vi "SkipForward.vi"(8 "error in (no error)":errorcluster, 10 "Message Queues in":T2, 11 "UI Refs in":T1) -> (0 "error out":errorcluster, 2 "Message Queues out":T2, 3 "UI Refs out":T1)   [LabVIEW 2015]
uses:
  support/Message Queue/All Message Queues.ctl
  support/Message Queue/Message Cluster.ctl
  Controls & Type Defs/UI Data.ctl
  Controls & Type Defs/SongDetails.ctl
  support/Message Queue/Enqueue Message (Single).vi
  support/Message Queue/Message Queue.lvlib
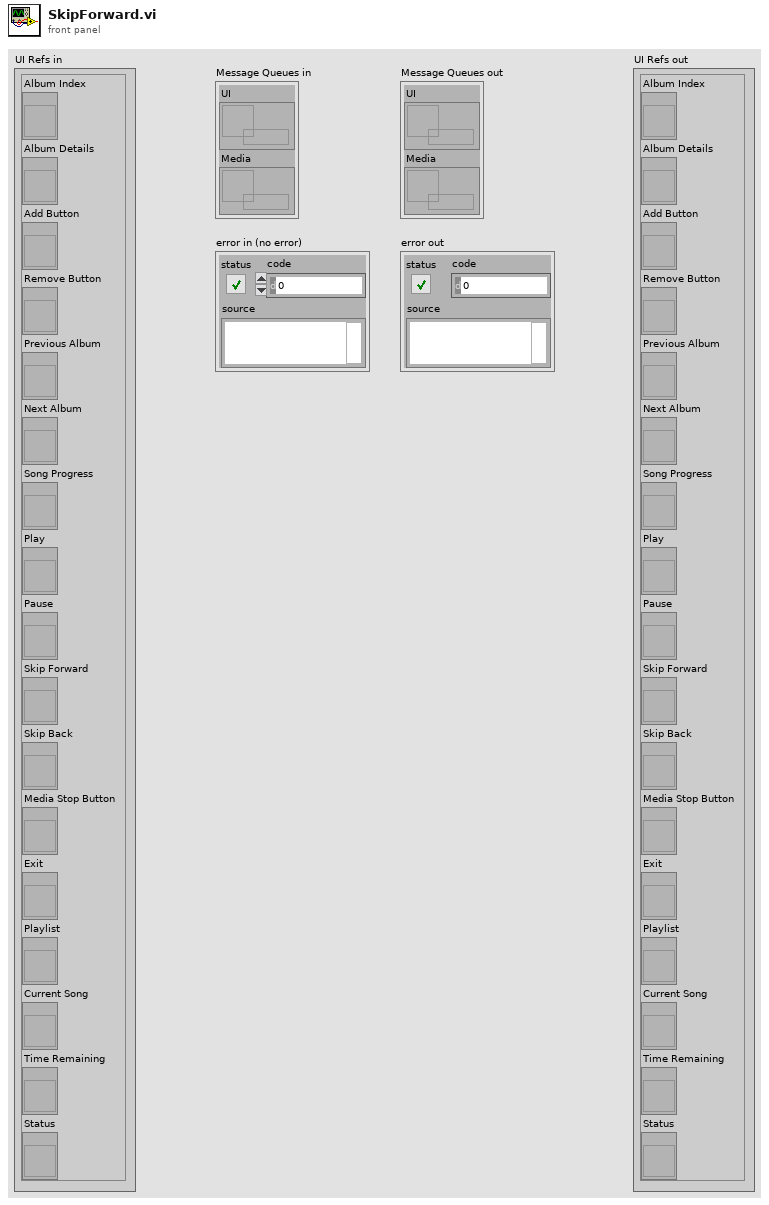
[diagram p1: front panel]
types:
  T1 = typedef "UI Data.ctl" = cluster{"Album Index":refnum<vi>, "Album Details":refnum<vi>, "Add Button":refnum<vi>, "Remove Button":refnum<vi>, "Previous Album":refnum<vi>, "Next Album":refnum<vi>, "Song Progress":refnum<vi>, "Play":refnum<vi>, "Pause ":refnum<vi>, "Skip Forward":refnum<vi>, "Skip Back":refnum<vi>, "Media Stop Button":refnum<vi>, "Exit":refnum<vi>, "Playlist":refnum<vi>, "Current Song":refnum<vi>, "Time Remaining":refnum<vi>, "Status":refnum<vi>}
  T2 = typedef "Message Queue.lvlib/All Message Queues.ctl" = cluster{"UI":refnum<queue>, "Media":refnum<queue>}
  T3 = typedef "SongDetails.ctl" = cluster{"Artist - Song Name":string, "Duration":string}
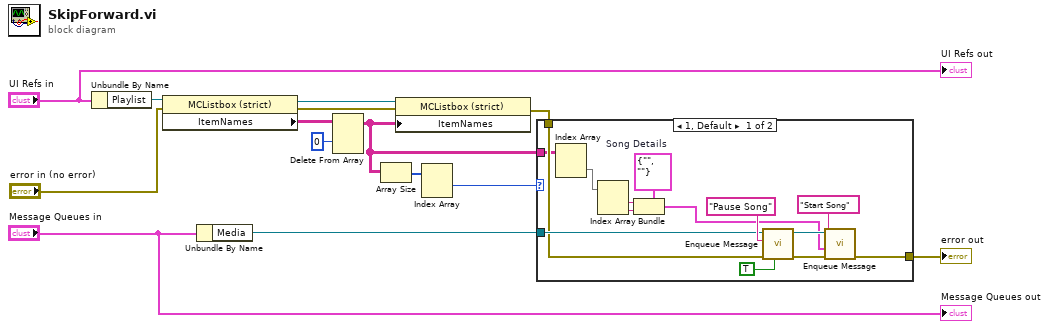
[diagram p0: block diagram]
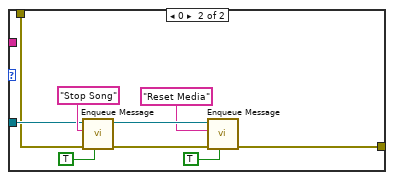
[diagram p2: hidden frame]
diagram:
  n1 = Unbundle By Name("UI Refs in") -> ("Playlist"=w14:refnum<vi>)
  n2 = property class="MCListbox (strict)"(reference=w14, error in="error in (no error)") -> (reference out=w11:refnum<vi>, error out=w10:errorcluster, "ItemNames"=w13:string[][])
  n3 = Unbundle By Name("Message Queues in") -> ("Media"=w9:refnum<queue>)
  n4 = Delete From Array(array=w13, index (row)=0) -> (array with subset deleted=w4:string[][])  [unwired: 2 in, 1 out]
  n5 = Array Size(array=w4) -> (size(s)=w3:i32[])
  n6 = property class="MCListbox (strict)"(reference=w11, error in=w10, "ItemNames"=w4) -> (error out=w8:errorcluster)  [unwired: 1 out]
  n7 = Index Array(array=w3) -> (element #1=w2:i32)  [unwired: 2 in, 1 out]
  n8 = case shown="1, Default" w2 {
    tunnel: w9 -> [w23 w36]
    tunnel: w8 -> [w22 w35]
    tunnel: [w18 w33] -> w7
    tunnel: w4 -> [w21 _]
    frame 1, Default {
      w28 = T3 {"Artist - Song Name"="", "Duration"=""}  # Song Details
      n9 = Index Array(array=w21) -> (element=w27:string[])  [unwired: 2 in]
      n10 = Index Array(array=w27) -> (element #1=w26:string, element #2=w25:string)  [unwired: 2 in]
      n11 = Bundle(cluster=w28, "Artist - Song Name"=w26, "Duration"=w25) -> (w15:T3)
      n12 = call-poly "Enqueue Message.vi"("Priority Message? (F)"=TRUE, "error in (no error)"=w22, "Message"="Pause Song", "Message Queue"=w23) -> ("error out"=w19:errorcluster, "dup Message Queue"=w20:refnum<queue>)  [unwired: 6 in]
      n13 = call-poly "Enqueue Message.vi"("error in (no error)"=w19, "Message Data"=w15, "Message"="Start Song", "Message Queue"=w20) -> ("error out"=w18:errorcluster)  [unwired: 6 in, 1 out]
    }
    frame 0 {
      n14 = call-poly "Enqueue Message.vi"("Priority Message? (F)"=TRUE, "error in (no error)"=w35, "Message"="Stop Song", "Message Queue"=w36) -> ("error out"=w34:errorcluster, "dup Message Queue"=w32:refnum<queue>)  [unwired: 6 in]
      n15 = call-poly "Enqueue Message.vi"("Priority Message? (F)"=TRUE, "error in (no error)"=w34, "Message"="Reset Media", "Message Queue"=w32) -> ("error out"=w33:errorcluster)  [unwired: 6 in, 1 out]
    }
  }
  "error out" <- w7
  "Message Queues out" <- "Message Queues in"
  "UI Refs out" <- "UI Refs in"
